vi "QueueAddTestCaseID.vi"(11 "test case ID":string) -> ()   [LabVIEW 2018]
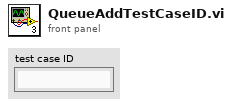
[diagram p1: front panel]
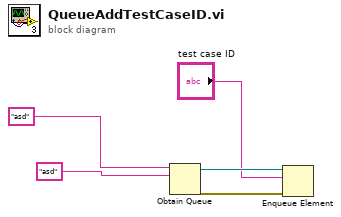
[diagram p0: block diagram]
diagram:
  n1 = Obtain Queue(name (unnamed)="asd", element data type="asd" ("name (unnamed)")) -> (queue out=w5:refnum<queue>, error out=w4:errorcluster)  [unwired: 3 in, 1 out]
  n2 = Enqueue Element(queue=w5, element="test case ID", error in (no error)=w4) -> ()  [unwired: 1 in, 3 out]
